vi "Robot Global Data.vi"() -> ()   [LabVIEW 2012]
doc: "This global VI can contain as many global variables as you need. Place a control on the panel, give it a good name. To read or write to it from a VI, drag the icon to the diagram of that VI. You can also drag from the project. Click on the node to change which global you access. You shouldn't have multiple locations writing to a global or it will cause a race-condition."
uses:
  <vilib>/Rock Robotics/WPI/Camera/WPI_CameraImageSize.ctl
  <vilib>/Rock Robotics/WPI/DriverStation/WPI_DriverStationRobotMode2.ctl
  <vilib>/Rock Robotics/WPI/Relay/WPI_RelayValue.ctl
panel:
  out "Flipper State":bool
  in  "Latch":dbl=25.0
  in  "Hold":dbl=85.0
  out "Enable Latch":bool
  out "OutLights":T1
  out "OutRight Flipper":dbl
  out "OutLeft Flipper":dbl
  out "OutRight Kicker":dbl
  out "OutLeft Kicker":dbl
  out "OutWheelB":dbl
  out "OutWheelF":dbl
  out "OutRotation":dbl
  out "OutExtension":dbl
  in  "POTPositions":T2={"Setpoint 1"=3.5, "Setpoint 2"=3.6, "Setpoint 3"=3.65, "Setpoint 4"=3.65, "RotLow"=3.4, "RotHigh"=3.8, "ExtLow"=1.74, "ExtHigh"=1.84}
  in  "ShooterServoPos":T3={"FlipperLeftUp"=30.0, "FlipperLeftDown"=115.0, "FlipperRightUp"=90.0, "FlipperRightDown"=90.0, "KickerLeftBack"=46.0, "KickerLeftForward"=100.0, "KickerRightBack"=124.0, "KickerRightForward"=68.0}
  in  "WheelBSpd":dbl=0.75
  in  "WheelFSpd":dbl=0.75
  in  "ExtDeadband":dbl=0.1
  in  "RotDeadband":dbl=0.1
  in  "YCoord":dbl
  in  "ManualRotate":dbl
  in  "ManualExtend":dbl
  in  "Shoot":bool
  in  "ShootEnableWheels":bool
  in  "VisionTrack":bool
  in  "Case":dbl
  in  "PTO Disabled":dbl=100.0
  in  "PTO Enabled":dbl=135.0
  out "Current File":dbl
  in  "Servo Positions":T4={"Right Servo High"=75.0, "Right Servo Mid"=92.0, "Right Servo Low"=110.0, "Left Servo High"=55.0, "Left Servo Mid"=75.0, "Left Servo Low"=90.0}
  out "Auton Array":dbl[][](array[numeric]) format="%0.3f"
  out "Auton Files":string[](array[string])
  out "Number of Auton Files":dbl
  in  "Robot Mode":T5
  in  "LED toggle rate (ms)":u32=20
  in  "image size":T6=enum."160x120"
  in  "Enable Vision":bool=TRUE
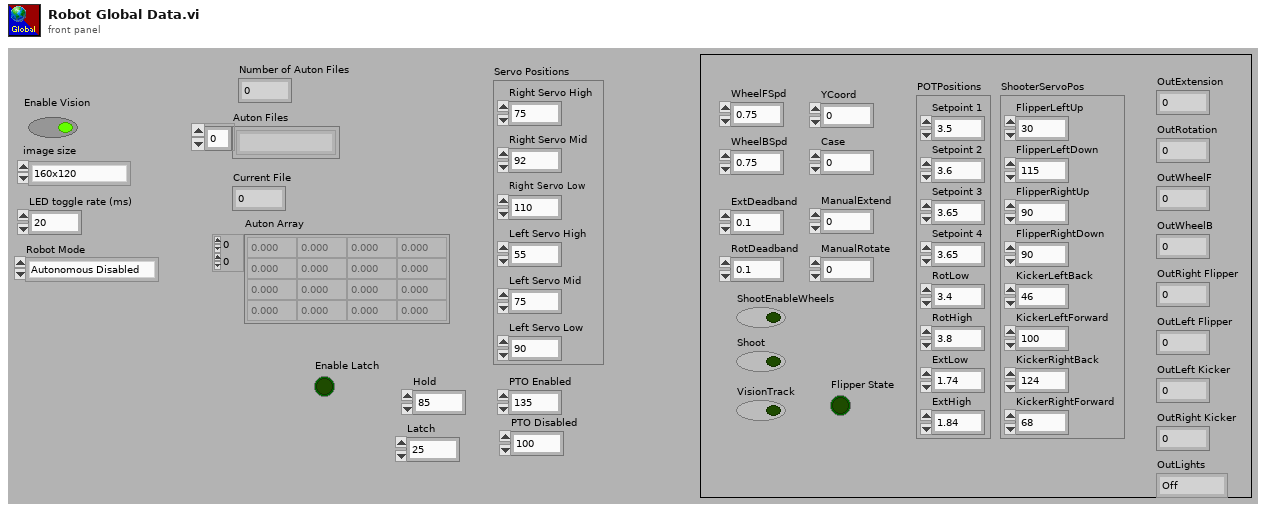
[diagram p1: front panel]
types:
  T1 = typedef "WPI_RelayValue.ctl" = enum16{"Off", "On", "Forward", "Reverse"}
  T2 = cluster{"Setpoint 1":dbl, "Setpoint 2":dbl, "Setpoint 3":dbl, "Setpoint 4":dbl, "RotLow":dbl, "RotHigh":dbl, "ExtLow":dbl, "ExtHigh":dbl}
  T3 = cluster{"FlipperLeftUp":dbl, "FlipperLeftDown":dbl, "FlipperRightUp":dbl, "FlipperRightDown":dbl, "KickerLeftBack":dbl, "KickerLeftForward":dbl, "KickerRightBack":dbl, "KickerRightForward":dbl}
  T4 = cluster{"Right Servo High":dbl, "Right Servo Mid":dbl, "Right Servo Low":dbl, "Left Servo High":dbl, "Left Servo Mid":dbl, "Left Servo Low":dbl}
  T5 = typedef "WPI_DriverStationRobotMode2.ctl" = enum16{"Autonomous Disabled", "Autonomous Enabled", "Teleop Disabled", "Teleop Enabled", "Timeout", "Finish", "Test Disabled", "Test Enabled"}
  T6 = typedef "WPI_CameraImageSize.ctl" = enum16{"640x480", "320x240", "160x120"}
diagram:
